vi "Read_adress-port.vi"(8 "error in (no error)":errorcluster, 11 "instrument in":refnum<class "instrument.lvclass">) -> (0 "error out":errorcluster, 1 "port number":i32, 2 "adress":string, 3 "instrument out":refnum<class "instrument.lvclass">)   [LabVIEW 2017, in "instrument.lvclass"]
doc: "instead of reading VISE-resource name, the VISE-resource name is split into a adress and port (separated by \":\" such as \"120.0.0.1:1069). This VI can be used if the instrument is connected bu UDP or TCPIP. There is no write_adress_port.vi. Just use the write_VISE-resource-name.vi."
uses:
  instrument.lvclass
  instrument.lvclass/instrument.ctl
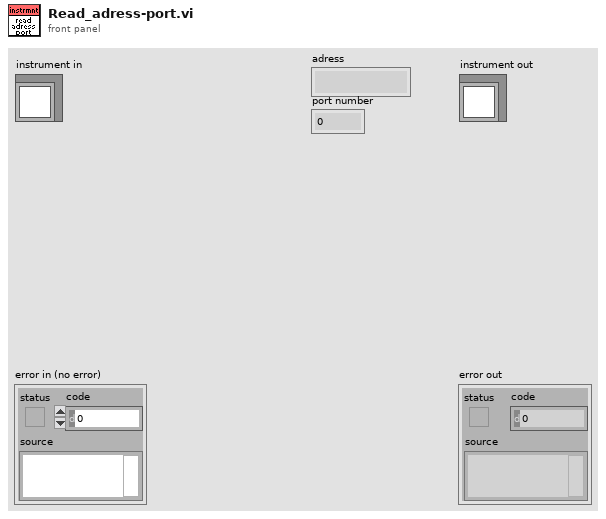
[diagram p1: front panel]
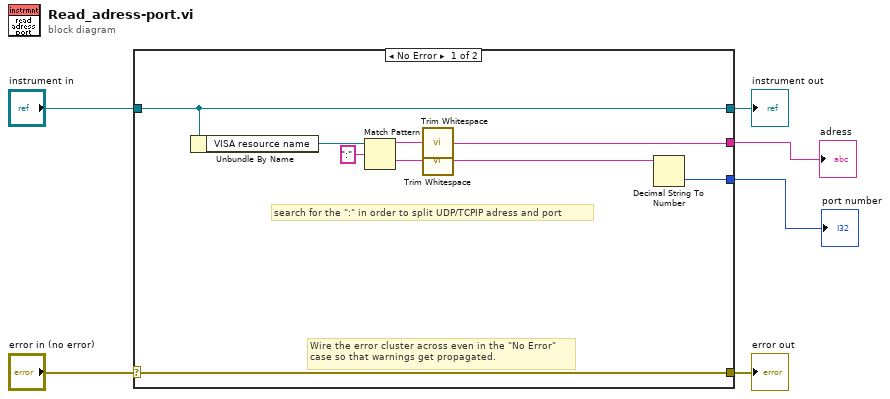
[diagram p0: block diagram]
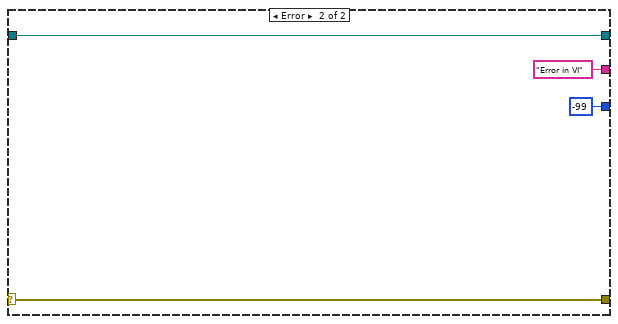
[diagram p2: hidden frame]
diagram:
  n1 = case shown="No Error" "error in (no error)" {
    selector: "error in (no error)" -> [w15 w19]
    tunnel: [w15 w19] -> w5
    tunnel: [w14 w18] -> w3
    tunnel: "instrument in" -> [w14 w18]
    tunnel: [w10 "Error in VI" ("trimmed string")] -> w2
    tunnel: [w7 -99] -> w1
    frame No Error {
      # "search for the \":\" in order to split UDP/TCPIP adress and port"
      # "Wire the error cluster across even in the \"No Error\"\ncase so that warnings get propagated."
      n2 = Unbundle By Name(w14) -> ("VISA resource name"=w13:refnum<visa-resource-name>)
      n3 = Match Pattern(string=w13, regular expression=":") -> (before substring=w11:string, after substring=w9:string)  [unwired: 1 in, 2 out]
      n4 = call <vilib>:"Trim Whitespace.vi"("string"=w11) -> ("trimmed string"=w10:string)  [unwired: 1 in]
      n5 = call <vilib>:"Trim Whitespace.vi"("string"=w9) -> ("trimmed string"=w8:string)  [unwired: 1 in]
      n6 = Decimal String To Number(string=w8) -> (number=w7:i32)  [unwired: 2 in, 1 out]
    }
    frame Error {
    }
  }
  "error out" <- w5
  "instrument out" <- w3
  "adress" <- w2
  "port number" <- w1
